vi "Configure Over Voltage.vi"(8 "error in (no error)":errorcluster, 10 "Set Overvoltage (0 V)":dbl format="%.2f", 11 "VISA resource name":refnum<visa-resource-name>) -> (0 "error out":errorcluster, 3 "VISA resource name out":refnum<visa-resource-name>)   [LabVIEW 2021, in "Sorensen M9A Series.lvlib"]
doc: "This VI sets the overvoltage protection trip point for the Sorensen power supply in Volts. The value must be within 0% and 110% of the maximum output voltage, VMAX. The default value on the power supply is 110% VMAX."
uses:
  Sorensen M9A Series.lvlib
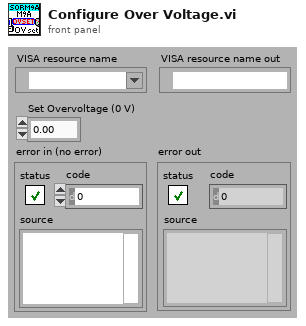
[diagram p1: front panel]
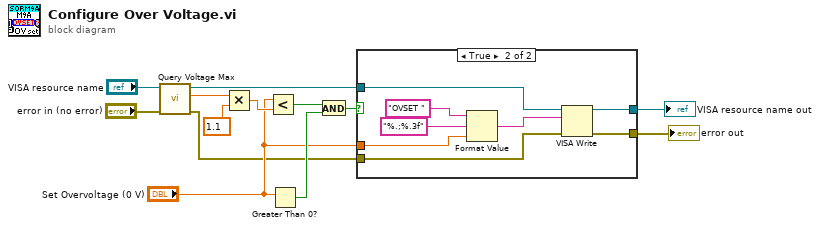
[diagram p0: block diagram]
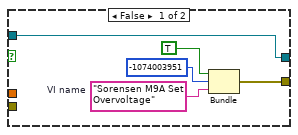
[diagram p2: hidden frame]
diagram:
  n1 = call "Query Voltage Max.vi"("error in (no error)"="error in (no error)", "VISA resource name"="VISA resource name") -> ("error out"=w2:errorcluster, "Voltage Max (V)"=w3:dbl, "VISA resource name out"=w4:refnum<visa-resource-name>)  [unwired: 7 in]
  n2 = Multiply(x=w3, y=1.1) -> (x*y=w7:dbl)
  n3 = Less?(x="Set Overvoltage (0 V)", y=w7) -> (x < y?=w8:bool)
  n4 = Greater Than 0?(x="Set Overvoltage (0 V)") -> (x > 0?=w9:bool)
  n5 = And(x=w8, y=w9) -> (x .and. y?=w10:bool)
  n6 = case shown="True" w10 {
    tunnel: [w15 w26] -> w13
    tunnel: [w14 w25] -> w12
    tunnel: "Set Overvoltage (0 V)" -> [_ w21]
    tunnel: w4 -> [w15 w20]
    tunnel: w2 -> [_ w19]
    frame False {
      w16 = "Sorensen M9A Set Overvoltage"  # VI name
      n7 = Bundle(TRUE, -1074003951, "VI name"=w16) -> (w14:cluster{bool, i32, "VI name":string})  [unwired: 1 in]
    }
    frame True {
      n8 = Format Value(string ("")="OVSET " ("data"), format string="%.;%.3f", value (0)=w21) -> (output string=w24:string)
      n9 = VISA Write(VISA resource name=w20, write buffer=w24, error in (no error)=w19) -> (VISA resource name out=w26:refnum<visa-resource-name>, error out=w25:errorcluster)  [unwired: 1 out]
    }
  }
  "error out" <- w12
  "VISA resource name out" <- w13
